vi "smoothing.vi"(5 "polynomial order":i32=9, 7 "side points":i32=19, 8 "Error In":errorcluster, 11 "Spectrum":i64[](array[numeric])) -> (0 "Error Out":errorcluster, 3 "Smoothed Spectrum":dbl[](array[numeric]))   [LabVIEW 2023]
uses:
  <vilib>/Analysis/1siggen.llb/Ramp Pattern by Samples.vi
  <vilib>/Analysis/3filter.llb/Savitzky-Golay Filter (DBL).vi
  <vilib>/Analysis/NI_AALBase.lvlib
panel:
  out "XY Graph":cluster{i64[], "Filtered X":dbl[]}[](graph)
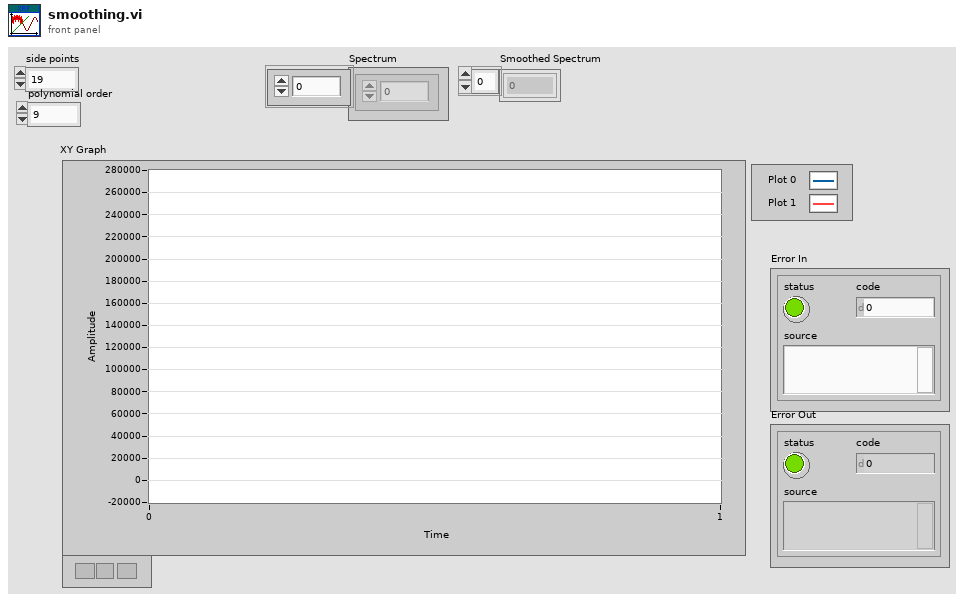
[diagram p1: front panel]
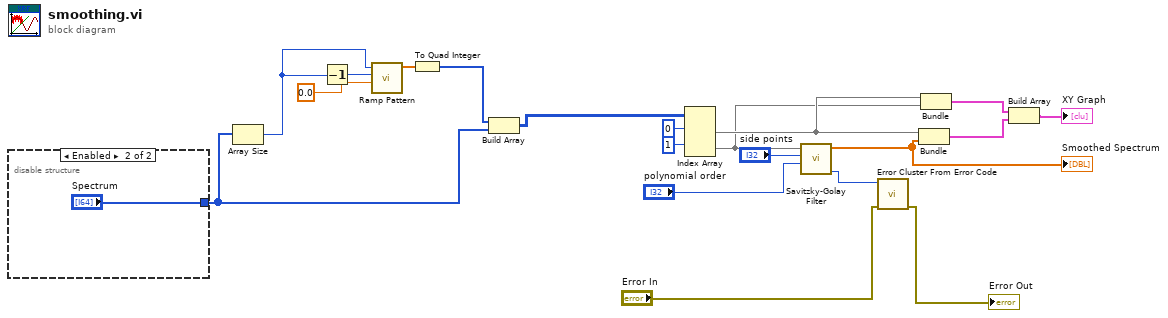
[diagram p0: block diagram]
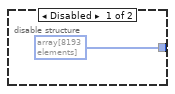
[diagram p2: hidden frame]
diagram:
  n1 = disable-structure shown="Enabled" {
    disable-tunnel: [i64[] array[8193 elements] ("subarray") "Spectrum"] -> w2
    frame Disabled {
    }
    frame Enabled {
    }
  }
  n2 = Array Size(array=w2) -> (size(s)=w1:i32)
  n3 = Decrement(x=w1) -> (x-1=w3:i32)
  n4 = call-poly <vilib>:"Ramp Pattern.vi"("start"=0.0, "end"=w3, "samples"=w1) -> ("Ramp Pattern"=w19:dbl[])  [unwired: 7 in, 1 out]
  n5 = To Quad Integer(1:w19) -> (0:w18:i64[])
  n6 = Build Array(w18, w2) -> (w17:i64[][])
  n7 = Index Array(array=w17, index (row) #1=0 ("index (row)"), index (row) #2=1 ("index (row)")) -> (element #1=w12:i64[], element #2=w10:i64[])  [unwired: 2 in]
  n8 = call-poly <vilib>:"Savitzky-Golay Filter.vi"("polynomial order"="polynomial order", "side points"="side points", "X"=w10) -> ("error"=w6:i32, "Filtered X"=w11:dbl[])  [unwired: 7 in]
  "Smoothed Spectrum" <- w11
  n9 = call <vilib>:"Error Cluster From Error Code.vi"("error in (no error)"="Error In", "error code (0)"=w6) -> ("error out"=→"Error Out":errorcluster)  [unwired: 7 in]
  n10 = Bundle(w12, "Filtered X"=w11) -> (w8:cluster{i64[], "Filtered X":dbl[]})  [unwired: 1 in]
  n11 = Bundle(w12, w10) -> (w9:cluster{i64[], i64[]})  [unwired: 1 in]
  n12 = Build Array(w9, w8) -> (→"XY Graph":cluster{i64[], "Filtered X":dbl[]}[])
